vi "Main_2.vi"() -> ()   [LabVIEW 2021]
uses:
  <vilib>/Utility/file.llb/Write Delimited Spreadsheet (string).vi
  Fonctions/Add_Library.lvlib
panel:
  in  "Exit":bool
  in  "Calculate":bool
  out "x+y":u64[](array[numeric])
  in  "y":u64[](array[numeric])=[1, 2, 3]
  in  "x":u64[](array[numeric])=[1, 2, 3]
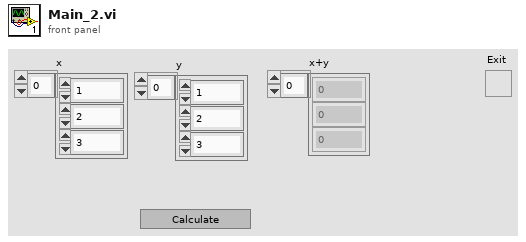
[diagram p1: front panel]
types:
  T1 = enum32{"invalid app kind", "Development System", "Run Time System", "Student Edition", "Embedded LabVIEW", "Evaluation", "Custom"}
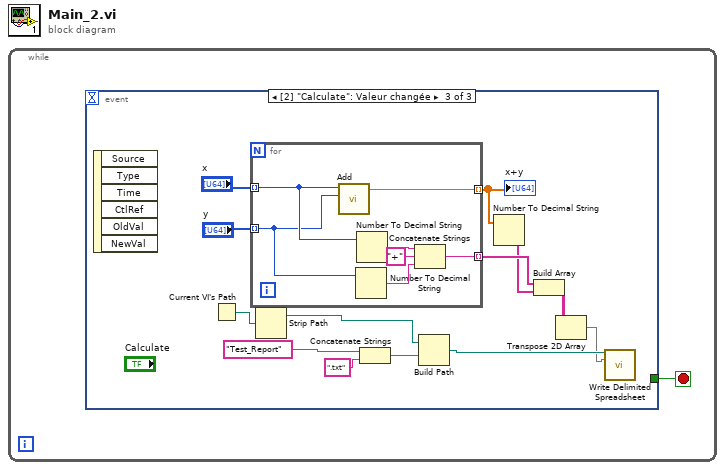
[diagram p0: block diagram]
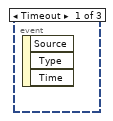
[diagram p2: hidden frame]
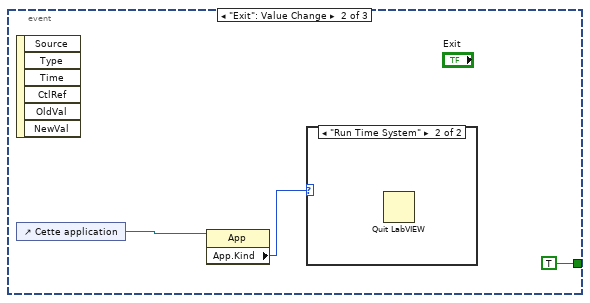
[diagram p3: hidden frame]
diagram:
  n1 = while {
    stop <- w1 stop-if-true
    n2 = event shown="[2] \"Calculate\": Valeur changée" {
      selector: _ -> [_ _ _]
      dyn-events: _ -> [_ _ _]
      timeout: _ -> [_ _ _]
      tunnel: [_ TRUE _] -> w1
      event Timeout {
        n3 = event-data() -> ()  [unwired: 1 in, 3 out]
      }
      event "Exit": Value Change {
        n4 = event-data() -> ()  [unwired: 1 in, 6 out]
        n5 = control-ref of="Cette application"() -> (w3:refnum<vi>)
        n6 = property class="App"(reference=w3) -> ("App.Kind"=w2:T1)  [unwired: 1 in, 2 out]
        n7 = case shown="\"Run Time System\"" w2 {
          frame "invalid app kind", Default {
          }
          frame "Run Time System" {
            n8 = Quit LabVIEW() -> ()  [unwired: 1 in]
          }
        }
      }
      event "Calculate": Value Change {
        n9 = event-data() -> ()  [unwired: 1 in, 6 out]
        n10 = Current VI's Path() -> (path=w10:path)
        n11 = for {
          tunnel: "x" -> [w23] mode=indexing
          tunnel: "y" -> [w22] mode=indexing
          tunnel: [w24] -> w15 mode=indexing
          tunnel: [w18] -> w14 mode=indexing
          n12 = call "Add.vi"("y"=w22, "x"=w23) -> ("x+y"=w24:dbl)  [unwired: 9 in]
          n13 = Number To Decimal String(number=w22) -> (decimal integer string=w19:string)  [unwired: 1 in]
          n14 = Number To Decimal String(number=w23) -> (decimal integer string=w21:string)  [unwired: 1 in]
          n15 = Concatenate Strings(w21, "+" ("chaîne"), w19) -> (w18:string)
        }
        "x+y" <- w15
        n16 = Strip Path(path=w10) -> (stripped path=w5:path)  [unwired: 1 out]
        n17 = Concatenate Strings("Test_Report" ("Report Path"), ".txt" ("chaîne")) -> (w9:string)
        n18 = Build Path(base path=w5, name or relative path=w9) -> (appended path=w8:path)
        n19 = Number To Decimal String(number=w15) -> (decimal integer string=w13:string[])  [unwired: 1 in]
        n20 = Build Array(w14, w13) -> (w7:string[][])
        n21 = Transpose 2D Array(2D array=w7) -> (transposed array=w6:string[][])
        n22 = call-poly <vilib>:"Write Delimited Spreadsheet.vi"("file path (dialog if empty)"=w8, "2D data"=w6) -> ()  [unwired: 12 in, 2 out]
      }
    }
  }
